vi "message_dialog_1.vi"(5 "display when parent not open? (F)":bool, 6 "name of caller in":string, 7 "display error? (F)":bool, 8 "Error in":errorcluster caption="Error in (no error)", 10 "flavour (warning)":enum16{"error", "warning", "message"}(ring)=enum."warning", 11 "text in":string) -> (0 "Error out":errorcluster)   [LabVIEW 2015]
uses:
  <vilib>/Utility/error.llb/DialogType.ctl
panel:
  in  "ok":bool
  out "text":string
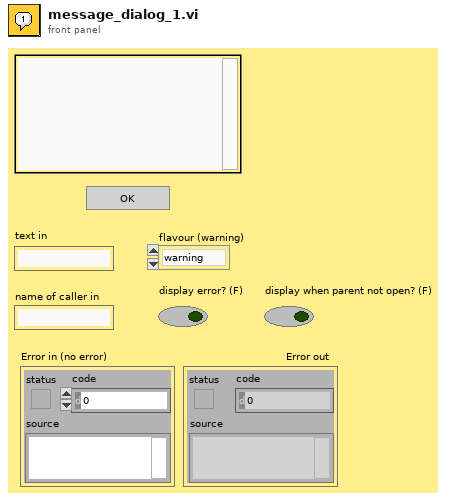
[diagram p1: front panel]
types:
  T1 = enum32{"Invalid", "Standard", "Closed", "Hidden", "Minimized", "Maximized"}
  T2 = typedef "DialogType.ctl" = u16
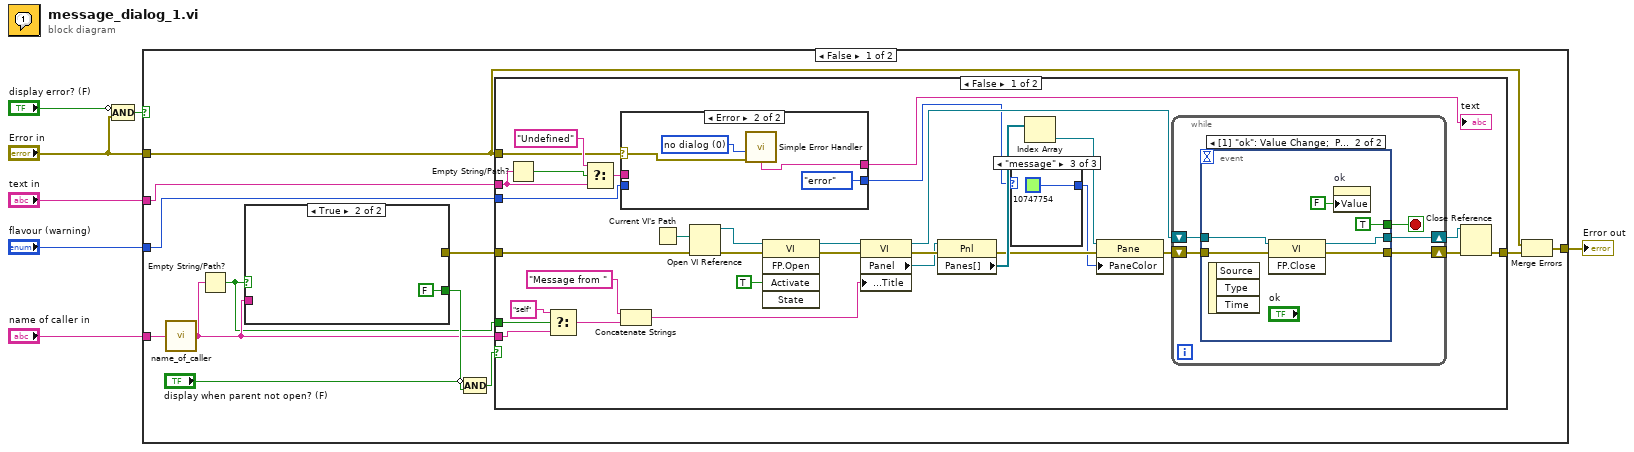
[diagram p0: block diagram]
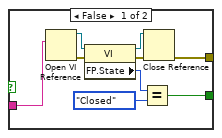
[diagram p2: hidden frame]
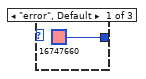
[diagram p4: hidden frame]
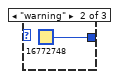
[diagram p5: hidden frame]
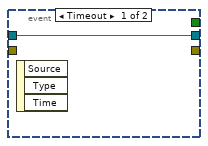
[diagram p6: hidden frame]
diagram:
  n1 = Compound Arithmetic op=AND(invert "display error? (F)", "Error in") -> (w3:bool)
  n2 = case shown="False" w3 {
    tunnel: "name of caller in" -> [w17 _]
    tunnel: [w13 w84] -> w2
    tunnel: "text in" -> [w19 _]
    tunnel: "Error in" -> [w15 w84]
    tunnel: "flavour (warning)" -> [w18 _]
    frame False {
      n3 = call "name_of_caller.vi"("name of caller in"=w17) -> ("name of caller out"=w9:string)  [unwired: 3 in]
      n4 = Empty String/Path?(string/path=w9) -> (empty?=w8:bool)
      n5 = case shown="True" w8 {
        tunnel: [w22 _] -> w16
        tunnel: [w21 FALSE] -> w12
        tunnel: w9 -> [w20 _]
        frame False {
          n6 = Open VI Reference(vi path=w20) -> (vi reference=w28:refnum<vi>, error out=w27:errorcluster)  [unwired: 5 in]
          n7 = property class="VI"(reference=w28, error in=w27) -> (reference out=w24:refnum<vi>, error out=w23:errorcluster, "FP.State"=w26:T1)
          n8 = Equal?(x=w26, y=T1."Closed" ("Front Panel Window:State")) -> (x = y?=w21:bool)
          n9 = Close Reference(reference=w24, error in (no error)=w23) -> (error out=w22:errorcluster)
        }
        frame True {
        }
      }
      n10 = Compound Arithmetic op=AND(invert "display when parent not open? (F)", w12) -> (w10:bool)
      n11 = case shown="False" w10 {
        tunnel: w19 -> [w43 _]
        tunnel: w18 -> [w42 _]
        tunnel: w15 -> [w34 _]
        tunnel: [w31 w83] -> w14
        tunnel: w9 -> [w33 _]
        tunnel: w16 -> [w32 w83]
        tunnel: w8 -> [w30 _]
        frame False {
          n12 = Empty String/Path?(string/path=w43) -> (empty?=w36:bool)
          n13 = Select(t="self", s=w30, f=w33) -> (s? t:f=w54:string)
          n14 = Select(t="Undefined" ("text in"), s=w36, f=w43) -> (s? t:f=w39:string)
          n15 = case shown="Error" w34 {
            selector: w34 -> [_ w66]
            tunnel: [w63 enum16{"error", "warning", "message"}."error" ("flavour (warning)")] -> w38
            tunnel: w42 -> [w63 _]
            tunnel: w39 -> [w62 _]
            tunnel: [w62 w65] -> w35
            frame No Error {
            }
            frame Error {
              w64 = T2 0 items=["no dialog", "OK message", "continue or stop message", "OK message + warnings", "continue/stop + warnings"] ("type of dialog (OK msg:1)")
              n16 = call <vilib>:"Simple Error Handler.vi"("type of dialog (OK msg:1)"=w64, "error in (no error)"=w66) -> ("message"=w65:string)  [unwired: 3 in, 4 out]
            }
          }
          "text" <- w35
          n17 = Concatenate Strings("Message from " ("string"), w54) -> (w55:string)
          n18 = Current VI's Path() -> (path=w61:path)
          n19 = Open VI Reference(vi path=w61, error in (no error)=w32) -> (vi reference=w51:refnum<vi>, error out=w49:errorcluster)  [unwired: 4 in]
          n20 = invoke class="VI" method="FP.Open"(reference=w51, error in=w49, "Activate"=TRUE) -> (reference out=w50:refnum<vi>, error out=w48:errorcluster)  [unwired: 2 in, 3 out]
          n21 = property class="VI"(reference=w50, error in=w48, "Front Panel.Title"=w55) -> (reference out=w47:refnum<vi>, error out=w57:errorcluster, "Panel"=w52:refnum<vi>)
          n22 = property class="Pnl"(reference=w52, error in=w57) -> (error out=w58:errorcluster, "Panes[]"=w60:refnum<vi>[])  [unwired: 1 out]
          n23 = case shown="\"message\"" w38 {
            tunnel: [u32 16747660 u32 16772748 u32 10747754] -> w41
            frame "error", Default {
            }
            frame "warning" {
            }
            frame "message" {
            }
          }
          n24 = Index Array(array=w60) -> (element=w59:refnum<vi>)  [unwired: 1 in]
          n25 = property class="Pane"(reference=w59, error in=w58, "PaneColor"=w41) -> (error out=w45:errorcluster)  [unwired: 1 out]
          n26 = while {
            shift-right: [w73] -> w46
            shift-left: w47 -> [w74]
            shift-right: [w71] -> w44
            shift-left: w45 -> [w72]
            stop <- w75 stop-if-true
            n27 = event shown="[1] \"ok\": Value Change;  Panel Close;  Key Down" {
              selector: _ -> [_ _]
              dyn-events: _ -> [_ _]
              timeout: _ -> [_ _]
              tunnel: [_ TRUE] -> w75
              tunnel: w74 -> [w76 w80]
              tunnel: [w76 w79] -> w73
              tunnel: w72 -> [_ w78]
              tunnel: [_ w77] -> w71
              event Timeout {
                n28 = event-data() -> ()  [unwired: 1 in, 3 out]
              }
              event "ok": Value Change; Panel Close; Key Down {
                n29 = event-data() -> ()  [unwired: 1 in, 3 out]
                n30 = invoke class="VI" method="FP.Close"(reference=w80, error in=w78) -> (reference out=w79:refnum<vi>, error out=w77:errorcluster)  [unwired: 1 in, 1 out]
                n31 = property on="ok" class="Bool (strict)"("Value"=FALSE ("ok")) -> ()  [unwired: 2 in, 2 out]
              }
            }
          }
          n32 = Close Reference(reference=w46, error in (no error)=w44) -> (error out=w31:errorcluster)
        }
        frame True {
        }
      }
      n33 = Merge Errors(w15, w14) -> (w13:errorcluster)
    }
    frame True {
    }
  }
  "Error out" <- w2
